vi "168xBSetVoltage_Current.vi"() -> ()   [LabVIEW 2015]
uses:
  <vilib>/Instr/_visa.llb/VISA Configure Serial Port (Instr).vi
panel:
  out "error out":errorcluster
  out "read buffer 2":string
  in  "Current":sgl min=0 max=30 step=0.1
  in  "VISA resource name":refnum<visa-resource-name>="COM5"
  in  "Voltage":sgl min=0 max=30 step=0.1
  out "read buffer":string
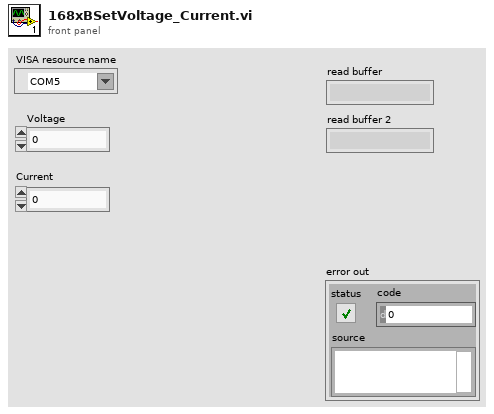
[diagram p1: front panel]
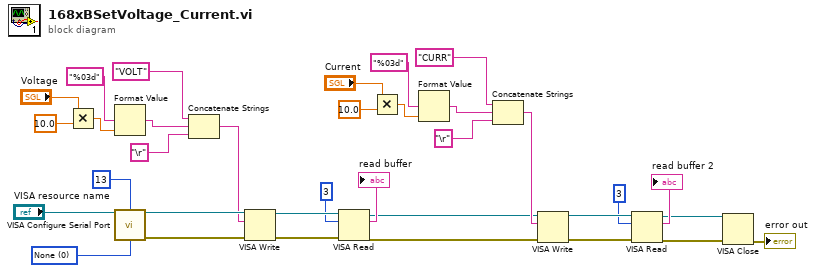
[diagram p0: block diagram]
diagram:
  w33 = u16 0 items=["None", "XON/XOFF", "RTS/CTS", "XON/XOFF & RTS/CTS", "DTR/DSR", "XON/XOFF & DTR/DSR"] ("flow control (0:none)")
  n1 = Multiply(x="Voltage", y=sgl 10.0) -> (x*y=w20:sgl)
  n2 = Format Value(format string="%03d", value (0)=w20) -> (output string=w19:string)  [unwired: 1 in]
  n3 = call-poly "VISA Configure Serial Port"("VISA resource name"="VISA resource name", "termination char\n(0xA = '\\n' = LF)"=u8 13 ("termination char\n(0xA = '\\n' = LF)"), "flow control (0:none)"=w33) -> ("VISA resource name out"=w27:refnum<visa-resource-name>, "error out"=w26:errorcluster)  [unwired: 11 in]
  n4 = Concatenate Strings("VOLT" ("write buffer"), w19, "\r" ("string")) -> (w23:string)
  n5 = VISA Write(VISA resource name=w27, write buffer=w23, error in (no error)=w26) -> (VISA resource name out=w31:refnum<visa-resource-name>, error out=w32:errorcluster)  [unwired: 1 out]
  n6 = VISA Read(VISA resource name=w31, byte count=u32 3, error in (no error)=w32) -> (VISA resource name out=w5:refnum<visa-resource-name>, read buffer=→"read buffer":string, error out=w4:errorcluster)  [unwired: 1 out]
  n7 = Multiply(x="Current", y=sgl 10.0) -> (x*y=w13:sgl)
  n8 = Format Value(format string="%03d", value (0)=w13) -> (output string=w12:string)  [unwired: 1 in]
  n9 = Concatenate Strings("CURR" ("write buffer"), w12, "\r" ("string")) -> (w6:string)
  n10 = VISA Write(VISA resource name=w5, write buffer=w6, error in (no error)=w4) -> (VISA resource name out=w9:refnum<visa-resource-name>, error out=w10:errorcluster)  [unwired: 1 out]
  n11 = VISA Read(VISA resource name=w9, byte count=u32 3, error in (no error)=w10) -> (VISA resource name out=w2:refnum<visa-resource-name>, read buffer=→"read buffer 2":string, error out=w1:errorcluster)  [unwired: 1 out]
  n12 = VISA Close(VISA resource name=w2, error in (no error)=w1) -> (error out=→"error out":errorcluster)
